vi "날짜시간문자열로포맷.vi"() -> ()   [LabVIEW 2014]
panel:
  out "날짜/시간 문자열":string
  out "웨이브폼 차트":dbl(graph)
  in  "정지":bool
  out "현재 시간":timestamp
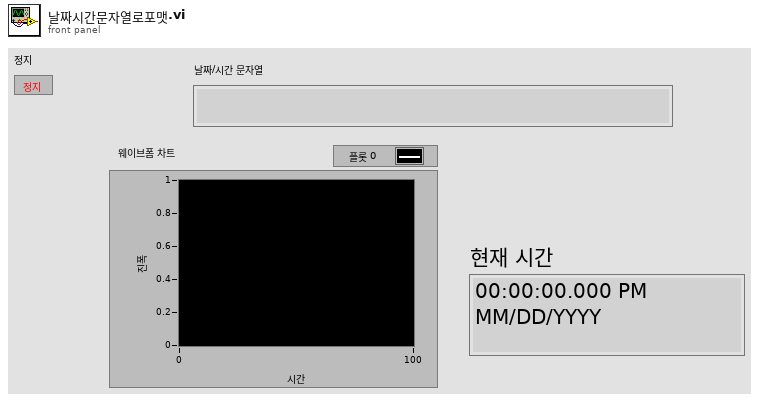
[diagram p1: front panel]
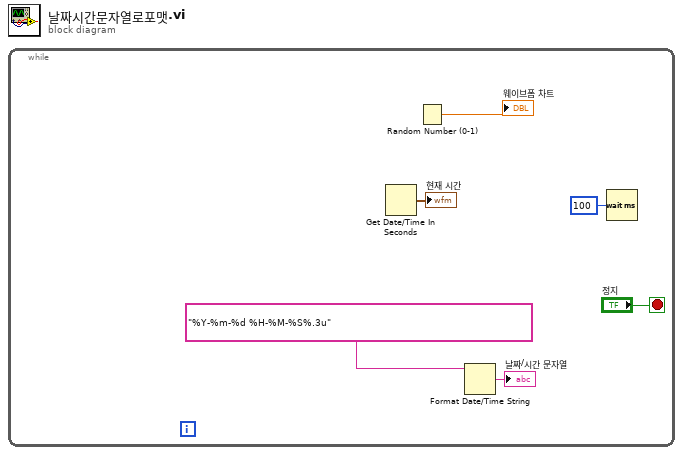
[diagram p0: block diagram]
diagram:
  n1 = while {
    stop <- "정지" stop-if-true
    n2 = Get Date/Time In Seconds() -> (seconds since 1Jan1904=→"현재 시간":timestamp)
    n3 = Random Number (0-1)() -> (number: 0 to 1=→"웨이브폼 차트":dbl)
    n4 = Format Date/Time String(time format string (%c)="%Y-%m-%d %H-%M-%S%.3u" ("시간 포맷 문자열 (%c)")) -> (date/time string=→"날짜/시간 문자열":string)  [unwired: 2 in]
    n5 = Wait (ms)(milliseconds to wait=u32 100 ("대기 시간(ms)")) -> ()  [unwired: 1 out]
  }
